vi "Laser Trainer.vi"() -> ()   [LabVIEW 2013]
uses:
  TrainerStates.ctl
panel:
  in  "Set Wavenumber":dbl=11828.99 format="%#_13g"
  out "Set Wavenumber":dbl format="%.4g"
  out "Trainer States":T1
  in  "Stop Button":bool
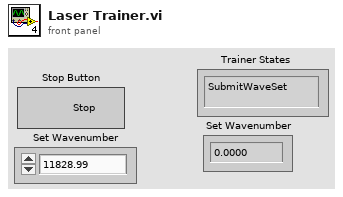
[diagram p1: front panel]
types:
  T1 = typedef "TrainerStates.ctl" = enum16{"SubmitWaveSet", "SubmitIsNew", "WaitFor RILISReady", "Wait while measurement", "reset isNew"}
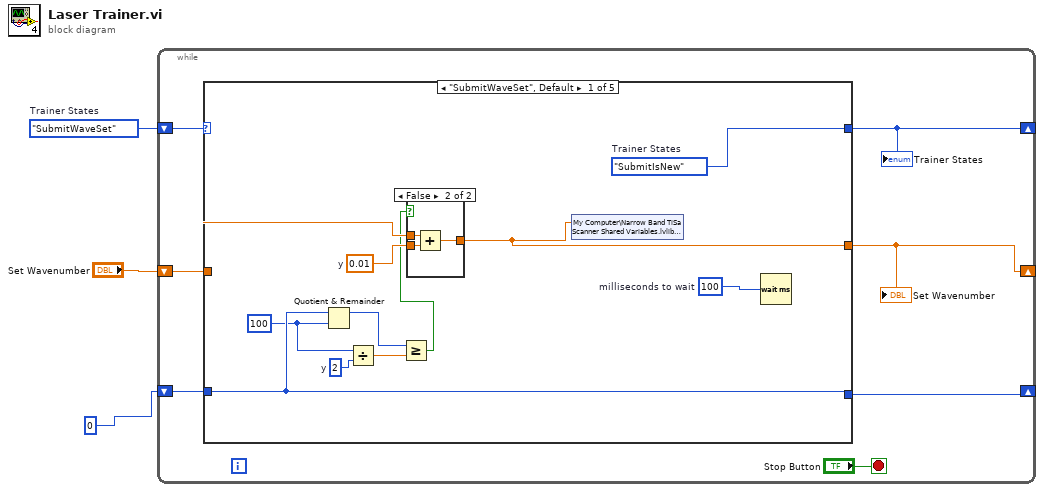
[diagram p0: block diagram]
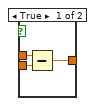
[diagram p2: hidden frame]
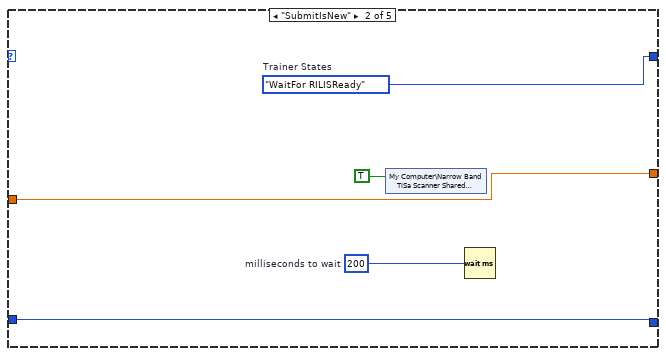
[diagram p3: hidden frame]
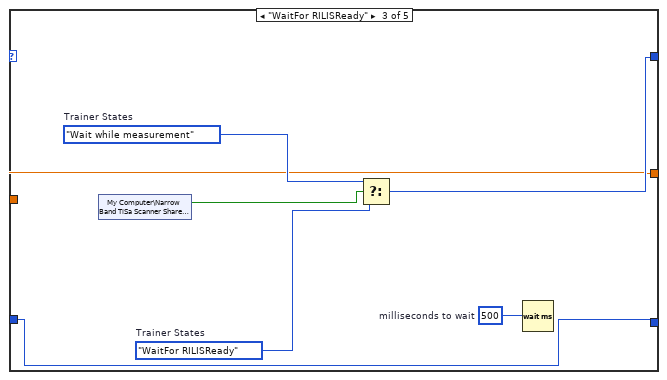
[diagram p4: hidden frame]
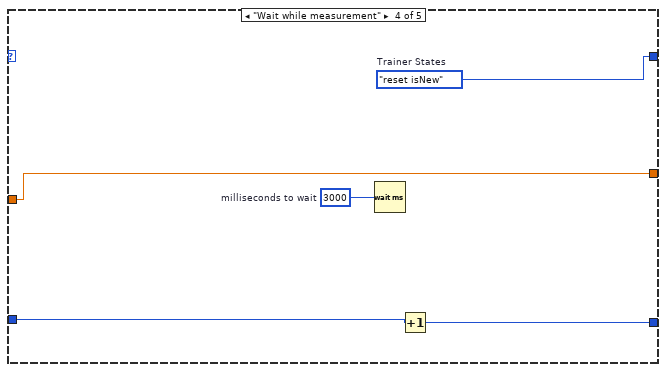
[diagram p5: hidden frame]
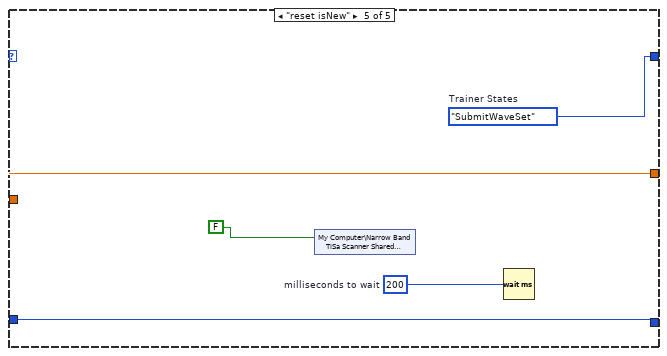
[diagram p6: hidden frame]
diagram:
  w3 = TrainerStates."SubmitWaveSet"  # Trainer States
  n1 = while {
    shift-right: [w9] -> _
    shift-left: w3 -> [w10]
    shift-right: [w6] -> _
    shift-left: "Set Wavenumber" -> [w7]
    shift-right: [w4] -> _
    shift-left: 0 -> [w5]
    stop <- "Stop Button" stop-if-true
    n2 = case shown="\"SubmitWaveSet\", Default" w10 {
      tunnel: [w20 w31 w37 w43 w48] -> w9
      tunnel: w7 -> [w19 w30 w34 w42 w47]
      tunnel: [w17 w30 w34 w42 w47] -> w6
      tunnel: w5 -> [w16 w29 w33 w41 w46]
      tunnel: [w16 w29 w33 w40 w46] -> w4
      frame "SubmitWaveSet", Default {
        w14 = 2  # y
        w15 = 100
        w18 = 0.01  # y
        w20 = TrainerStates."SubmitIsNew"  # Trainer States
        w21 = u32 100  # milliseconds to wait
        n3 = Quotient & Remainder(x=w16, y=w15) -> (x-y*floor(x/y)=w13:i32)  [unwired: 1 out]
        n4 = Divide(x=w15, y=w14) -> (x/y=w12:dbl)
        n5 = Greater Or Equal?(x=w13, y=w12) -> (x >= y?=w11:bool)
        n6 = case shown="False" w11 {
          tunnel: w19 -> [w24 w27]
          tunnel: w18 -> [w23 w26]
          tunnel: [w22 w25] -> w17
          frame True {
            n7 = Subtract(x=w24, y=w23) -> (x-y=w22:dbl)
          }
          frame False {
            n8 = Add(x=w27, y=w26) -> (x+y=w25:dbl)
          }
        }
        n9 = shared-variable "My Computer\\Narrow Band TiSa Scanner Shared Variables.lvlib\\waveSet_test"(w17) -> ()  [unwired: 1 in, 1 out]
        n10 = Wait (ms)(milliseconds to wait=w21) -> ()  [unwired: 1 out]
      }
      frame "SubmitIsNew" {
        w28 = u32 200  # milliseconds to wait
        w31 = TrainerStates."WaitFor RILISReady"  # Trainer States
        n11 = shared-variable "My Computer\\Narrow Band TiSa Scanner Shared Variables.lvlib\\isNew_test"(TRUE) -> ()  [unwired: 1 in, 1 out]
        n12 = Wait (ms)(milliseconds to wait=w28) -> ()  [unwired: 1 out]
      }
      frame "WaitFor RILISReady" {
        w35 = u32 500  # milliseconds to wait
        w36 = TrainerStates."WaitFor RILISReady"  # Trainer States
        w38 = TrainerStates."Wait while measurement"  # Trainer States
        n13 = shared-variable "My Computer\\Narrow Band TiSa Scanner Shared Variables.lvlib\\isOK_test"() -> (w39:bool)  [unwired: 1 in, 1 out]
        n14 = Select(t=w38, s=w39, f=w36) -> (s? t:f=w37:T1)
        n15 = Wait (ms)(milliseconds to wait=w35) -> ()  [unwired: 1 out]
      }
      frame "Wait while measurement" {
        w43 = TrainerStates."reset isNew"  # Trainer States
        w44 = u32 3000  # milliseconds to wait
        n16 = Wait (ms)(milliseconds to wait=w44) -> ()  [unwired: 1 out]
        n17 = Increment(x=w41) -> (x+1=w40:i32)
      }
      frame "reset isNew" {
        w45 = u32 200  # milliseconds to wait
        w48 = TrainerStates."SubmitWaveSet"  # Trainer States
        n18 = shared-variable "My Computer\\Narrow Band TiSa Scanner Shared Variables.lvlib\\isNew_test"(FALSE) -> ()  [unwired: 1 in, 1 out]
        n19 = Wait (ms)(milliseconds to wait=w45) -> ()  [unwired: 1 out]
      }
    }
    "Trainer States" <- w9
    "Set Wavenumber" <- w6
  }
